vi "CONVERT HEX TO VOLTAGE.vi"(10 "SUPPLY RANGE":T1, 11 "HEX STRING":string) -> (2 "x/y":dbl[unit])   [LabVIEW 2018]
uses:
  Control 1.ctl
  <vilib>/Utility/error.llb/whitespace.ctl
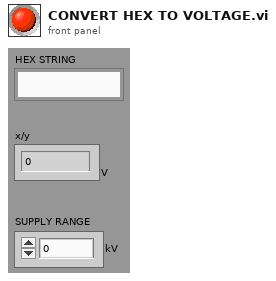
[diagram p1: front panel]
types:
  T1 = typedef "Control 1.ctl" = dbl[unit]
  T2 = typedef "whitespace.ctl" = u16
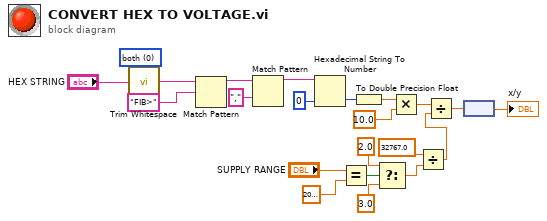
[diagram p0: block diagram]
diagram:
  w22 = T2 0 items=["both", "start of string", "end of string"] ("location (both)")
  n1 = call <vilib>:"Trim Whitespace.vi"("string"="HEX STRING", "location (both)"=w22) -> ("trimmed string"=w21:string)
  n2 = Match Pattern(string=w21, regular expression="FIB>") -> (before substring=w19:string)  [unwired: 1 in, 3 out]
  n3 = Match Pattern(string=w19, regular expression=",") -> (before substring=w3:string)  [unwired: 1 in, 3 out]
  n4 = Hexadecimal String To Number(string=w3, default (0uL)=u16 0 ("default (0 U32)")) -> (number=w1:u16)  [unwired: 1 in, 1 out]
  n5 = Equal?(x="SUPPLY RANGE", y=dbl[unit] 20000.0) -> (x = y?=w11:bool)
  n6 = To Double Precision Float(number=w1) -> (double precision float=w6:dbl)
  n7 = Select(t=2.0, s=w11, f=3.0) -> (s? t:f=w8:dbl)
  n8 = Multiply(x=w6, y=10.0) -> (x*y=w15:dbl)
  n9 = Divide(x=32767.0, y=w8) -> (x/y=w7:dbl)
  n10 = Divide(x=w15, y=w7) -> (x/y=w5:dbl)
  n11 = node(w5) -> (→"x/y":dbl[unit])
